vi "DETERMINE_PHASE.vi"() -> ()   [LabVIEW 2015]
uses:
  GS_COMMANDS.ctl
  PHASES.ctl
panel:
  out "PHASES":T1
  in  "GS_COMMAND":T2
  in  "VEL":dbl
  in  "STANDBY_SPEED":dbl
  in  "PUSHER_LS2":bool
  in  "PUSHER_LS1":bool
  in  "REAR_X_POSITION":dbl
  in  "ACC":dbl
  in  "LIFTED":bool
  in  "TESTS_SUCCESFUL":bool
  in  "stop":bool
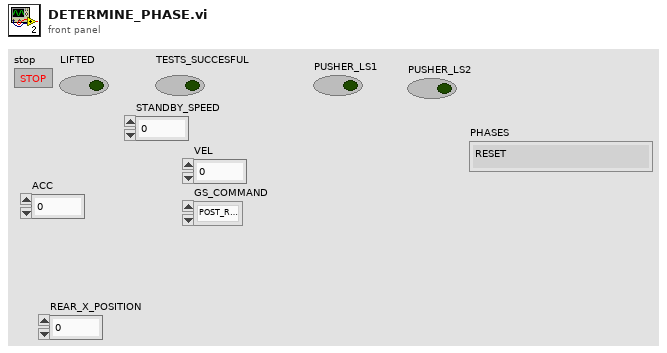
[diagram p1: front panel]
types:
  T1 = typedef "PHASES.ctl" = enum16{"RESET", "TEST", "PRE_RUN", "PUSHER_INTERLOCK", "FLIGHT", "POST_RUN"}
  T2 = typedef "GS_COMMANDS.ctl" = enum16{"POST_RUN_TO_PRE_RUN"}
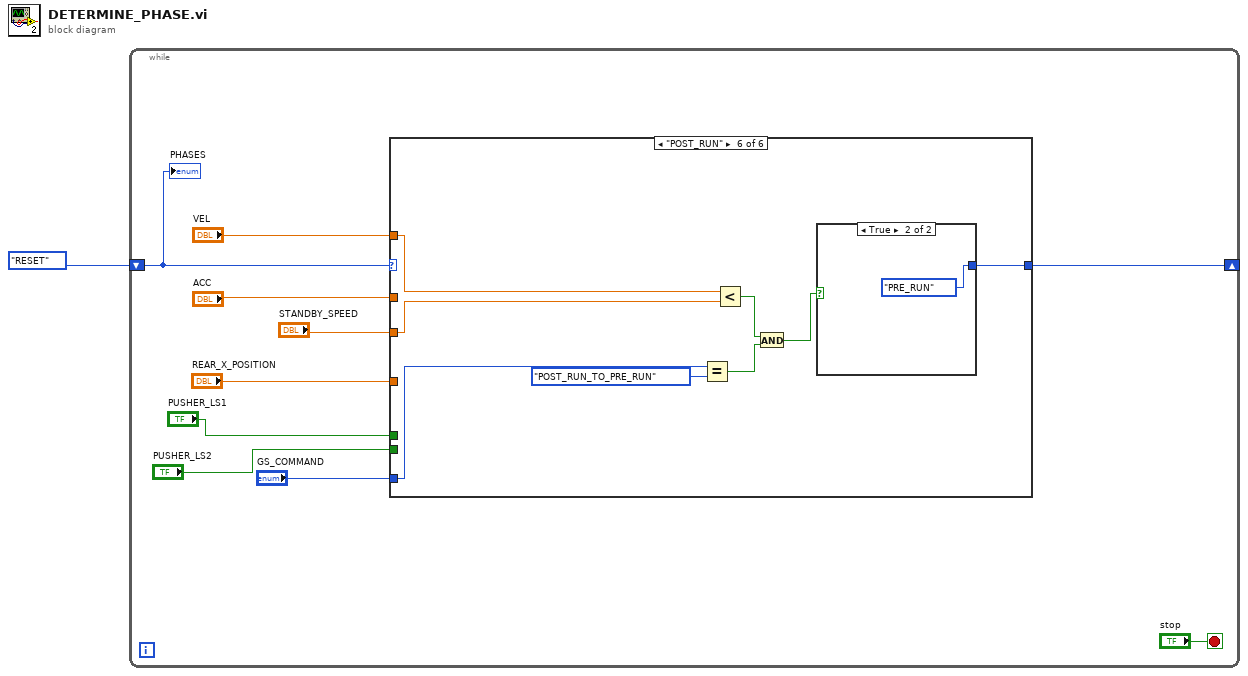
[diagram p0: block diagram]
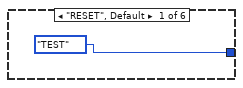
[diagram p2: hidden frame]
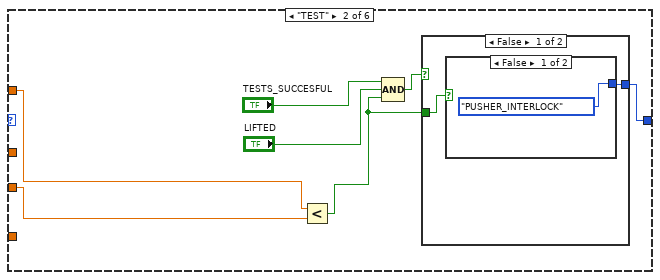
[diagram p3: hidden frame]
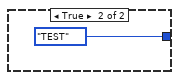
[diagram p4: hidden frame]
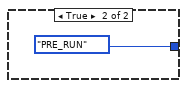
[diagram p5: hidden frame]
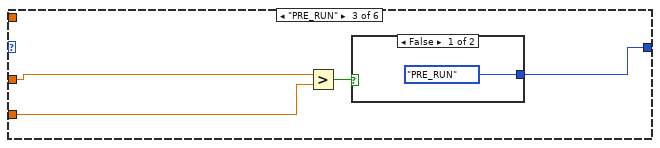
[diagram p6: hidden frame]
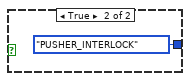
[diagram p7: hidden frame]
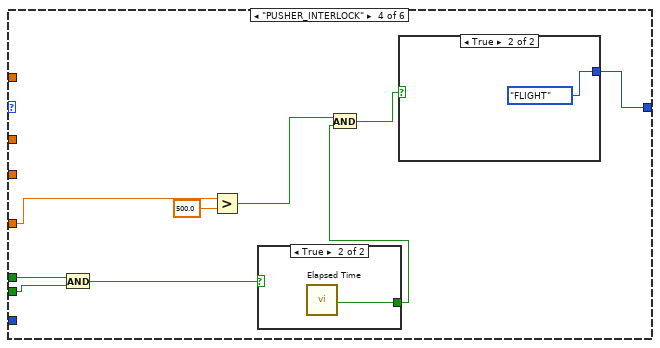
[diagram p8: hidden frame]
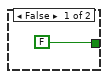
[diagram p9: hidden frame]
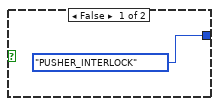
[diagram p10: hidden frame]
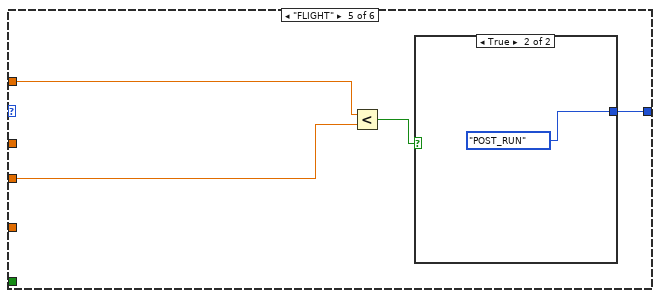
[diagram p11: hidden frame]
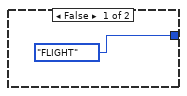
[diagram p12: hidden frame]
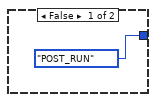
[diagram p13: hidden frame]
diagram:
  n1 = while {
    shift-right: [w5] -> _
    shift-left: PHASES."RESET" ("PHASES") -> [w4]
    stop <- "stop" stop-if-true
    n2 = case shown="\"POST_RUN\"" w4 {
      tunnel: [PHASES."TEST" ("PHASES") w19 w27 w39 w45 w50] -> w5
      tunnel: "ACC" -> [_ _ w26 _ _ _]
      tunnel: "REAR_X_POSITION" -> [_ _ _ w38 _ _]
      tunnel: "STANDBY_SPEED" -> [_ w14 w25 _ w47 w56]
      tunnel: "VEL" -> [_ w13 _ _ w46 w57]
      tunnel: "GS_COMMAND" -> [_ _ _ _ _ w55]
      tunnel: "PUSHER_LS1" -> [_ _ _ w32 _ _]
      tunnel: "PUSHER_LS2" -> [_ _ _ w31 _ _]
      frame "RESET", Default {
      }
      frame "TEST" {
        n3 = Less?(x=w13, y=w14) -> (x < y?=w15:bool)
        n4 = Compound Arithmetic op=AND("TESTS_SUCCESFUL", "LIFTED", w15) -> (w16:bool)
        n5 = case shown="False" w16 {
          tunnel: [w21 PHASES."PRE_RUN" ("PHASES")] -> w19
          tunnel: w15 -> [w20 _]
          frame False {
            n6 = case shown="False" w20 {
              tunnel: [PHASES."PUSHER_INTERLOCK" ("PHASES") PHASES."TEST" ("PHASES")] -> w21
              frame False {
              }
              frame True {
              }
            }
          }
          frame True {
          }
        }
      }
      frame "PRE_RUN" {
        n7 = Greater?(x=w26, y=w25) -> (0:w28:bool)
        n8 = case shown="False" w28 {
          tunnel: [PHASES."PRE_RUN" ("PHASES") PHASES."PUSHER_INTERLOCK" ("PHASES")] -> w27
          frame False {
          }
          frame True {
          }
        }
      }
      frame "PUSHER_INTERLOCK" {
        n9 = And(x=w32, y=w31) -> (x .and. y?=w36:bool)
        n10 = Greater?(x=w38, y=500.0) -> (0:w35:bool)
        n11 = case shown="True" w36 {
          tunnel: [FALSE w41] -> w34
          frame False {
          }
          frame True {
            n12 = call "Elapsed Time"() -> ("Time has Elapsed"=w41:bool)  [unwired: 12 in, 7 out]
          }
        }
        n13 = And(x=w35, y=w34) -> (x .and. y?=w33:bool)
        n14 = case shown="True" w33 {
          tunnel: [PHASES."PUSHER_INTERLOCK" ("PHASES") PHASES."FLIGHT" ("PHASES")] -> w39
          frame False {
          }
          frame True {
          }
        }
      }
      frame "FLIGHT" {
        n15 = Less?(x=w46, y=w47) -> (x < y?=w44:bool)
        n16 = case shown="True" w44 {
          tunnel: [PHASES."FLIGHT" ("PHASES") PHASES."POST_RUN" ("PHASES")] -> w45
          frame False {
          }
          frame True {
          }
        }
      }
      frame "POST_RUN" {
        n17 = Equal?(x=w55, y=GS_COMMANDS."POST_RUN_TO_PRE_RUN") -> (x = y?=w52:bool)
        n18 = Less?(x=w57, y=w56) -> (x < y?=w53:bool)
        n19 = And(x=w53, y=w52) -> (x .and. y?=w51:bool)
        n20 = case shown="True" w51 {
          tunnel: [PHASES."POST_RUN" ("PHASES") PHASES."PRE_RUN" ("PHASES")] -> w50
          frame False {
          }
          frame True {
          }
        }
      }
    }
    "PHASES" <- w4
  }
